vi "ダミーデータ作成.vi"() -> ()   [LabVIEW 2014]
doc: "シミュレートされた入力信号の平均化されたパワースペクトルを計算します。このサンプルは、RMS平均、ベクトル平均、ピークホールド、平均の数といったさまざまな平均モードを計測用に指定します。これらの平均化パラメータの影響を主にノイズの視点で確認できます。基本派成分を低下させないようにノイズを軽減するには、ベクトル平均化でトリガが必要です。ハニング窓やフラットトップ窓など、この測定に使用する窓タイプを指定することができます。"
uses:
  <vilib>/measure/NI_MABase.lvlib
  <vilib>/measure/NI_MAPro.lvlib
  <vilib>/measure/maspectr.llb/FFT Power Spectrum and PSD for 1 Chan.vi
panel:
  in  "再生ボタン":bool
  in  "平均化パラメータ":T1={"平均化モード"=enum."RMS averaging", "加重モード"=enum."Exponential", "平均数"=10} {"平均数" min=1}
  in  "窓":i32(ring)=1 items=["四角", "ハニング", "ハミング", "ブラックマン・ハリス", "完全ブラックマン", "ブラックマン", "フラットトップ", "4項ブラックマン・ハリス ", "7項ブラックマン・ハリス", "低サイドローブ", "ブラックマン・ナットール", "三角", "バートレット・ハニング", "ボーマン", "パーゼン", "ウェルチ", "カイザー", "ドルフ・チェビシェフ", "ガウス"]
  in  "停止":bool
  in  "dB":bool=TRUE
  in  "正弦波振幅":dbl(slide)=1.0 min=0.0 scale=0.0..10.0
  in  "トリガ":bool
  in  "正弦周波数":dbl(knob)=2409.6320656484827 scale=0.0..10000.0 scale format="%0.0f"
  in  "平均化を再開":bool
  out "完了平均数":dbl=27.0
  out "線形平均化完了":bool=TRUE
  out "パワースペクトル":cluster{"f0":dbl, "df":dbl, "magnitude":dbl[]}(graph)
  # "概要: FFTパワースペクトルとPSDVIの使用法を説明します。\n要件: LabVIEW開発システム\n手順:\n1.VIを実行します。\n2.正弦周波数を変更し、平均化されたパワースペクトルの結果の変化を観察します。\n3.平均化パラメータを変更し、さまざまなFFT平均化モードや加重モードを使用してみます。\n4.平均化モードが「ベクトル平均化」の場合、正弦波信号が各レコードで同じ位相になるようにトリガをONにする必要があります。\n5.停止をクリックしてVIを停止します。"
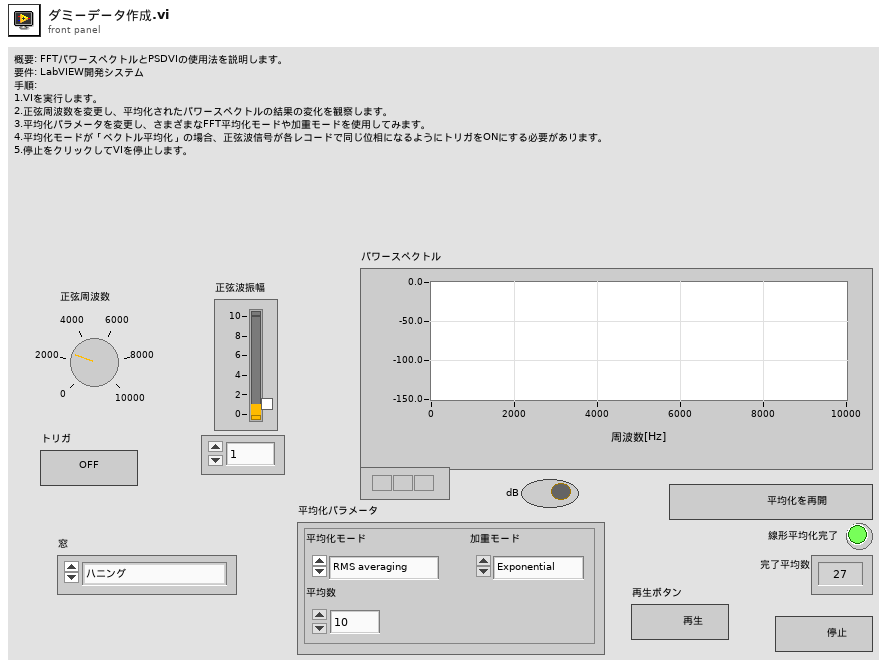
[diagram p1: front panel]
types:
  T1 = cluster{"平均化モード":enum16{"No averaging", "Vector averaging", "RMS averaging", "Peak hold"}, "加重モード":enum16{"Linear", "Exponential"}, "平均数":u32}
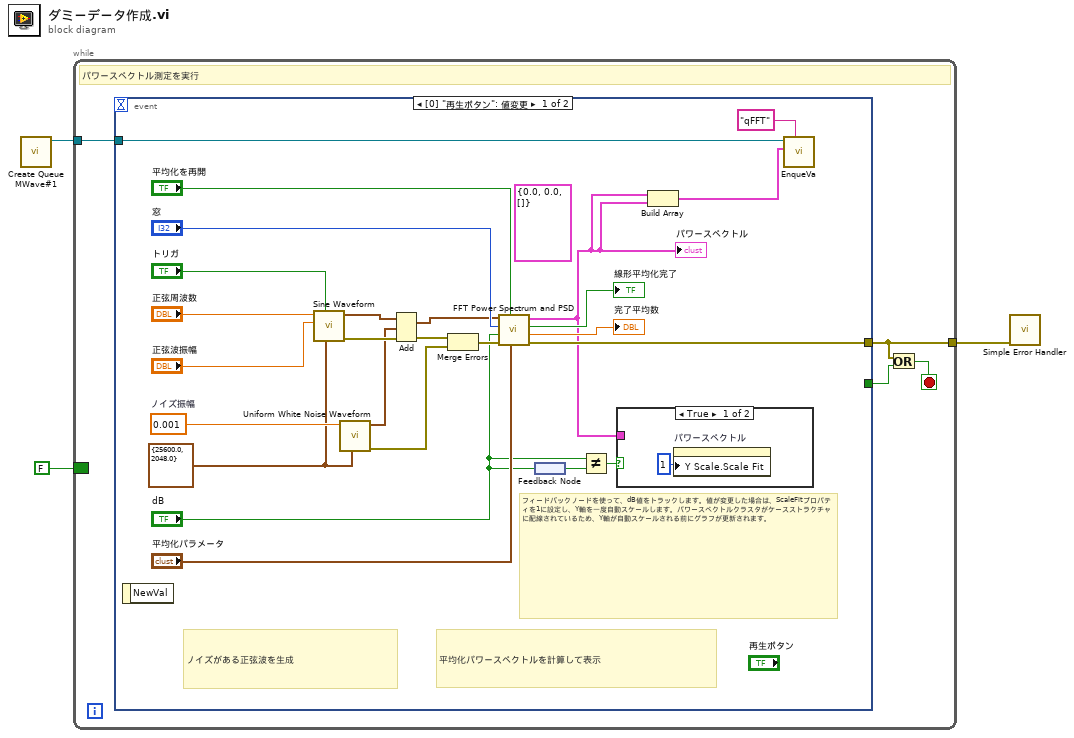
[diagram p0: block diagram]
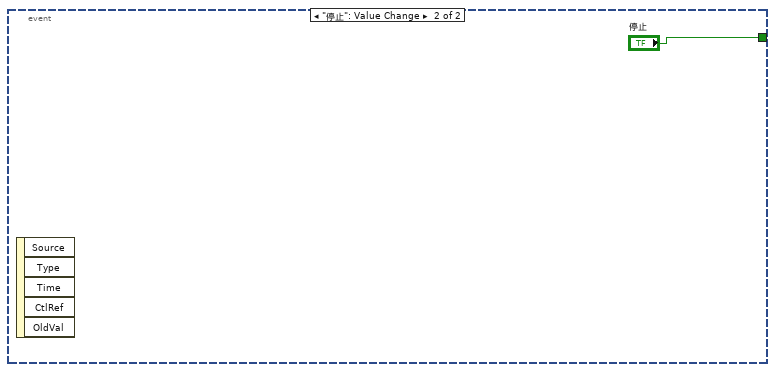
[diagram p3: hidden frame]
diagram:
  n1 = call "Create Queue MWave#1.vi"() -> ("queMWave#1"=w1:refnum<queue>)  [unwired: 10 in, 1 out]
  n2 = while {
    tunnel: [w7] -> w3
    border: FALSE ("dB") -> [_]
    tunnel: w1 -> [w4]
    stop <- w5 stop-if-true
    # "パワースペクトル測定を実行"
    n3 = event shown="[0] \"再生ボタン\": 値変更" {
      selector: _ -> [_ _]
      dyn-events: _ -> [_ _]
      timeout: _ -> [_ _]
      tunnel: [w14 _] -> w7
      tunnel: [_ "停止"] -> w6
      tunnel: w4 -> [w10 _]
      event "再生ボタン": Value Change {
        (unwired) cluster{"f0":dbl, "df":dbl, "magnitude":dbl[]} {"f0"=0.0, "df"=0.0, "magnitude"=[]} ("Power Spectrum / PSD")
        w20 = cluster{"Fs":dbl, "#s":dbl} {"Fs"=25600.0, "#s"=2048.0} ("sampling info")
        w22 = 0.001  # ノイズ振幅
        # "フィードバックノードを使って、dB値をトラックします。値が変更した場合は、ScaleFitプロパティを1に設定し、Y軸を一度自動スケールします。パワースペクトルクラスタがケースストラクチャに配線されているため、Y軸が自動スケールされる前にグラフが更新されます。"
        # "平均化パワースペクトルを計算して表示"
        # "ノイズがある正弦波を生成"
        n4 = event-data() -> ()  [unwired: 1 in, 1 out]
        n5 = call <vilib>:"Sine Waveform.vi"("sampling info"=w20, "reset signal"="トリガ", "amplitude"="正弦波振幅", "frequency"="正弦周波数") -> ("error out"=w32:errorcluster, "signal out"=w24:waveform(dbl))  [unwired: 6 in]
        n6 = call <vilib>:"Uniform White Noise Waveform.vi"("sampling info"=w20, "amplitude"=w22) -> ("error out"=w17:errorcluster, "signal out"=w23:waveform(dbl))  [unwired: 8 in]
        n7 = Add(1:w23, 2:w24, 4:w32) -> (0:w25:waveform(dbl), 3:w15:errorcluster)
        n8 = Merge Errors(w15, w17) -> (w16:errorcluster)
        n9 = call-poly <vilib>:"FFT Power Spectrum and PSD.vi"("averaging parameters"="平均化パラメータ", "restart averaging (F)"="平均化を再開", "error in (no error)"=w16, "dB On (F)"="dB", "window"="窓", "time signal"=w25) -> ("error out"=w14:errorcluster, "averages completed"=→"完了平均数":dbl, "averaging done"=→"線形平均化完了":bool, "Power Spectrum / PSD"=w11:cluster{"f0":dbl, "df":dbl, "magnitude":dbl[]})  [unwired: 2 in]
        "パワースペクトル" <- w11
        n10 = feedback #1() -> (w12:bool)
        n11 = feedback-in #1("dB") -> ()
        n12 = Not Equal?(x="dB", y=w12) -> (x != y?=w21:bool)
        n13 = case shown="TRUE" w21 {
          tunnel: w11 -> [_ _]
          frame True {
            n14 = property on="パワースペクトル" class="WFGraph （指定）"("Y Scale.Scale Fit"=u8 1) -> ()  [unwired: 2 in, 2 out]
          }
          frame False {
          }
        }
        n15 = Build Array(w11, w11) -> (w8:cluster{"f0":dbl, "df":dbl, "magnitude":dbl[]}[])
        n16 = call "EnqueVa.vi"("コマンド"="qFFT", "バリアント"=w8, "queVariant"=w10) -> ()  [unwired: 6 in, 3 out]
      }
      event "停止": Value Change {
        n17 = event-data() -> ()  [unwired: 1 in, 5 out]
      }
    }
    n18 = Or(x=w7, y=w6) -> (x .or. y?=w5:bool)
  }
  n19 = call <vilib>:"Simple Error Handler.vi"("error in (no error)"=w3) -> ()  [unwired: 4 in, 5 out]
